vi "IFilterOpen.vi"() -> (1 "PRIORLib.IFilterOut":refnum<k7>, 2 "error out":errorcluster)   [LabVIEW 2011]
panel:
  in  "PRIORLib.IFilterIn":refnum<k7>
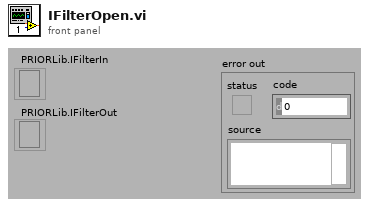
[diagram p1: front panel]
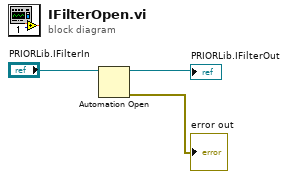
[diagram p0: block diagram]
diagram:
  n1 = Automation Open(Automation Refnum="PRIORLib.IFilterIn") -> (Automation Refnum=→"PRIORLib.IFilterOut":refnum<k7>, error out=→"error out":errorcluster)  [unwired: 3 in]
